vi "UDBox5G_sample.vi"() -> ()   [LabVIEW 2022 SP3]
uses:
  C:/Users/Ron_Wang/Documents/Projects/bbox-api/example/UDBox/LabVIEW/BBoxAPI.dll
  BBoxAPI.dll
panel:
  in  "SetState":i32[](array[numeric])=[0, 1, 1, 0, 0, 0, 0, 0, 0]
  in  "Bandwidth (KHz)":u32=200000 step=100000
  in  "IF Frequency (KHz)":u32=2000000 step=100000
  in  "RF Frequency (KHz)":u32=28000000 step=100000
  in  "UD Frequency (KHz)":u32=26000000 step=100000
  out "Init":i32(ring)=13 items=["OK"=0, "WARNING"=1, "ERROR"=2, "NO_RESPONSE"=3, "ERROR_GET_SN"=10, "ERROR_DEV_TYPE"=11, "ERROR_INIT_OBJECT"=12, "ERROR_DEV_NOT_INIT"=13, "ERROR_METHOD_NOT_FOUND"=14, "ERROR_REFLECTION"=15, "ERROR_POWER"=16, "ERROR_NETWORK_NOT_INIT"=20, "ERROR_NETWORK_INIT"=21, "ERROR_NETWORK_CONNECT_TIMEOUT"=22, "ERROR_DISCONNECT"=23, "ERROR_SOCKET"=24, "ERROR_SEND_CMD"=25, "ERROR_RESP_CMD"=26, "ERROR_DEV_COUNT_ZERO"=30, "ERROR_CMD"=40, "ERROR_CMD_INIT"=41, "ERROR_BF_AAKIT"=100, "ERROR_BF_NO_AAKIT"=101, "ERROR_BF_CALI_PATH"=102, "ERROR_BF_BEAMXY"=103, "ERROR_BF_GEN"=104, "ERROR_BF_TRMODE"=105, "STATUS_BF_LOAD_CALI_INCOMPLTE"=106, "ERROR_BF_LOAD_CALI_PARSE_FAILED"=107, "ERROR_FREQ_EQUATION"=250, "ERROR_PLO_CRC"=251, "WARNING_HARMONIC"=252, "ERROR_HARMONIC_BLOCK"=253]
  out "SN":string
  out "GetState":i32[](array[numeric])
  out "ScanningDevice":string[](array[string])
  # "UD state array, the following is index description\n0: PLO Lock (0: Unlock, 1: Lock)\n1: Ch1 (0: Disable, 1:Enable)\n2: Ch2 (0: Disable, 1:Enable)\n3: 10MHz output (0: Disable, 1:Enable)\n4: 100MHz output (0: Disable, 1:Enable)\n5: 100MHz source (0:Internal, 1:External)\n6: 100MHz LED( 0:Off, 1:White, 2:Blue)\n7: 5V output (0: Disable, 1:Enable)\n8: 9V output (0: Disable, 1:Enable)\n9: error code"
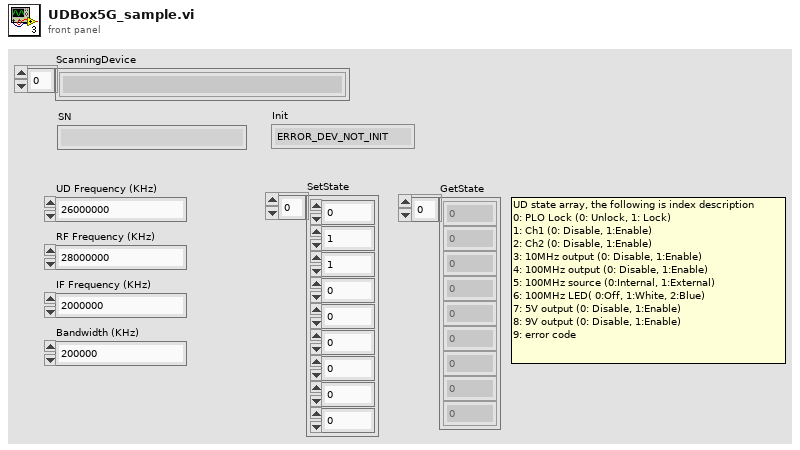
[diagram p1: front panel]
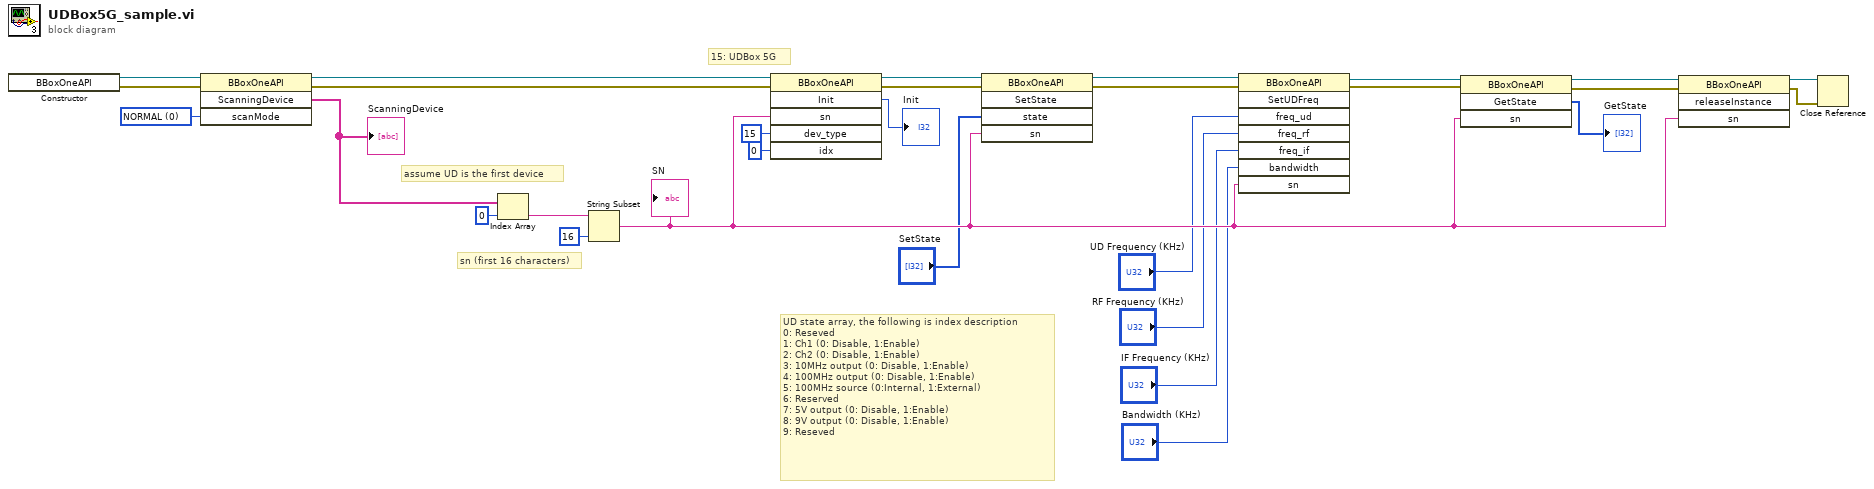
[diagram p0: block diagram]
diagram:
  w8 = 0 items=["NORMAL", "FAST", "ETH_DISABLE"] ("scanMode")
  # "15: UDBox 5G"
  # "UD state array, the following is index description\n0: Reseved\n1: Ch1 (0: Disable, 1:Enable)\n2: Ch2 (0: Disable, 1:Enable)\n3: 10MHz output (0: Disable, 1:Enable)\n4: 100MHz output (0: Disable, 1:Enable)\n5: 100MHz source (0:Internal, 1:External)\n6: Reserved\n7: 5V output (0: Disable, 1:Enable)\n8: 9V output (0: Disable, 1:Enable)\n9: Reseved"
  # "assume UD is the first device"
  # "sn (first 16 characters)"
  n1 = constructor class="BBoxOneAPI"() -> (reference out=w28:refnum<k24>, error out=w22:errorcluster)  [unwired: 3 in, 1 out]
  n2 = invoke class="BBoxOneAPI" method="ScanningDevice"(reference=w28, error in=w22, "scanMode"=w8) -> (reference out=w29:refnum<k24>, error out=w21:errorcluster, "ScanningDevice"=w27:string[])  [unwired: 1 in, 1 out]
  "ScanningDevice" <- w27
  n3 = Index Array(array=w27, index=0) -> (element=w25:string)
  n4 = String Subset(string=w25, length (rest)=16 ("length (rest)")) -> (substring=w7:string)  [unwired: 1 in]
  "SN" <- w7
  n5 = invoke on="Invoke Node" class="BBoxOneAPI" method="Init"(reference=w29, error in=w21, "sn"=w7, "dev_type"=15, "idx"=0) -> (reference out=w23:refnum<k24>, error out=w20:errorcluster, "Init"=→"Init":i32)  [unwired: 1 in, 3 out]
  n6 = invoke class="BBoxOneAPI" method="SetState"(reference=w23, error in=w20, "state"="SetState", "sn"=w7) -> (reference out=w19:refnum<k24>, error out=w15:errorcluster)  [unwired: 1 in, 3 out]
  n7 = invoke class="BBoxOneAPI" method="SetUDFreq"(reference=w19, error in=w15, "freq_ud"="UD Frequency (KHz)", "freq_rf"="RF Frequency (KHz)", "freq_if"="IF Frequency (KHz)", "bandwidth"="Bandwidth (KHz)", "sn"=w7) -> (reference out=w17:refnum<k24>, error out=w16:errorcluster)  [unwired: 1 in, 6 out]
  n8 = invoke class="BBoxOneAPI" method="GetState"(reference=w17, error in=w16, "sn"=w7) -> (reference out=w13:refnum<k24>, error out=w14:errorcluster, "GetState"=→"GetState":i32[])  [unwired: 1 in, 1 out]
  n9 = invoke class="BBoxOneAPI" method="releaseInstance"(reference=w13, error in=w14, "sn"=w7) -> (reference out=w11:refnum<k24>, error out=w12:errorcluster)  [unwired: 1 in, 2 out]
  n10 = Close Reference(reference=w11, error in (no error)=w12) -> ()  [unwired: 1 out]
